vi "Demo - Simple Use.vi"() -> ()   [LabVIEW 2013, in "GOLPI library.lvlib"]
uses:
  GOLPI library.lvlib
panel:
  in  "command":string="sin(3)\n\n"
  out "GNU Octave version":string
  out "exit code":i32
  out "error out":errorcluster
  out "read buffer":string
  in  "Octave binary directory":path=path "C:/Program Files/Octave-3.6.2/bin"
  in  "Working directory":path=path "C:/"
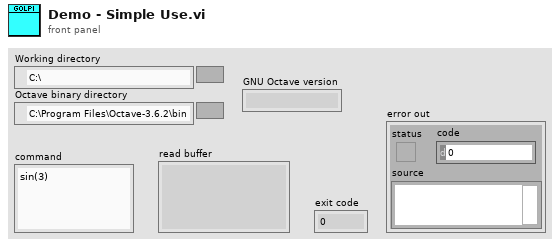
[diagram p1: front panel]
types:
  T1 = typedef "LV Process.lvlibp/Pipe Handle.ctl" = cluster{"lv_proc.dll file path":path, "process instance handle":u32[]}
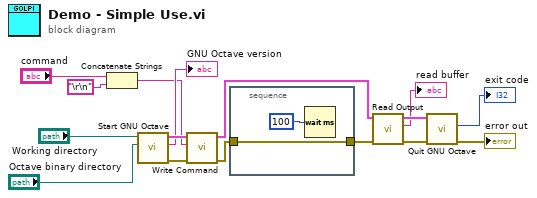
[diagram p0: block diagram]
diagram:
  n1 = Concatenate Strings("command", "\r\n") -> (w1:string)
  n2 = call "Start GNU Octave.vi"("Octave binary directory"="Octave binary directory", "Working directory"="Working directory") -> ("error out"=w11:errorcluster, "GNU Octave version"=→"GNU Octave version":string, "pipe out"=w14:T1)  [unwired: 6 in, 1 out]
  n3 = call "Write Command.vi"("error in"=w11, "command"=w1, "pipe in"=w14) -> ("error out"=w10:errorcluster, "pipe out"=w13:T1)  [unwired: 7 in]
  n4 = stacked-sequence {
    tunnel: [w17] -> w9
    tunnel: w10 -> [w17]
    frame #0 {
      n5 = Wait (ms)(milliseconds to wait=u32 100) -> ()  [unwired: 1 out]
    }
  }
  n6 = call "Read Output.vi"("error in"=w9, "pipe in"=w13) -> ("error out"=w7:errorcluster, "read buffer"=→"read buffer":string, "pipe out"=w12:T1)  [unwired: 6 in, 1 out]
  n7 = call "Quit GNU Octave.vi"("error in"=w7, "pipe in"=w12) -> ("error out"=→"error out":errorcluster, "exit code"=→"exit code":i32)  [unwired: 8 in]
